vi "ReadConfig.vi"() -> ()   [LabVIEW 2021]
uses:
  <vilib>/Utility/file.llb/Read Delimited Spreadsheet (DBL).vi
panel:
  out "all rows":dbl[][](array[numeric])
  out "array":dbl[][](array[numeric])
  in  "text to write":string="test"
  out "error out":errorcluster
  out "text read":string
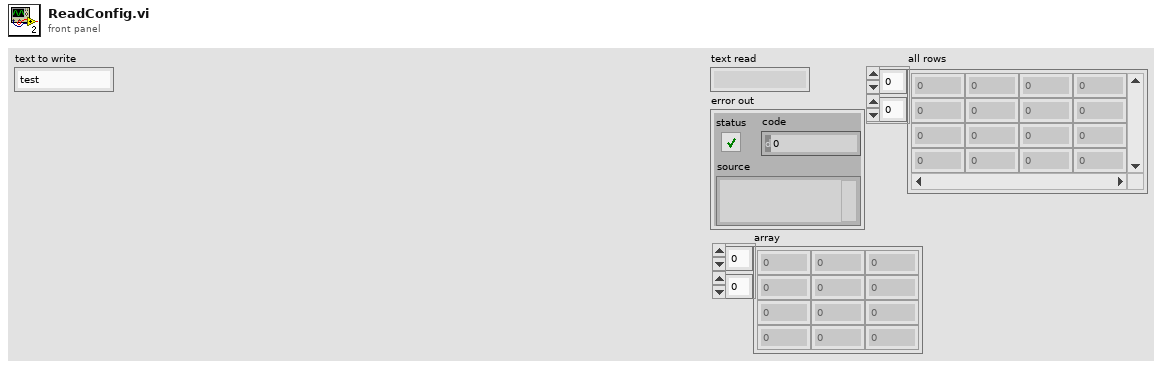
[diagram p1: front panel]
types:
  T1 = enum16{"open", "replace", "create", "open or create", "replace or create", "replace or create with confirmation"}
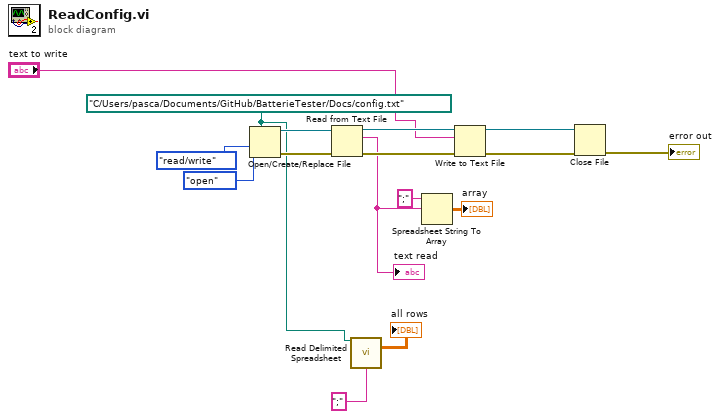
[diagram p0: block diagram]
diagram:
  w3 = path "C:/Users/pasca/Documents/GitHub/BatterieTester/Docs/config.txt"
  n1 = Open/Create/Replace File(file path (use dialog)=w3, operation (0:open)=T1."open", access (0:read/write)=enum16{"read/write", "read-only", "write-only"}."read/write") -> (refnum out=w14:refnum<file>, error out=w13:errorcluster)  [unwired: 3 in, 1 out]
  n2 = Read from Text File(file (use dialog)=w14, error in=w13) -> (refnum out=w9:refnum<file>, text=w6:string, error out=w12:errorcluster)  [unwired: 2 in, 1 out]
  "text read" <- w6
  n3 = call-poly <vilib>:"Read Delimited Spreadsheet.vi"("file path (dialog if empty)"=w3, "delimiter (\\t)"=";" ("delimiter (\\t)")) -> ("all rows"=→"all rows":dbl[][])  [unwired: 8 in, 5 out]
  n4 = Spreadsheet String To Array(format string=";", spreadsheet string=w6) -> (array=→"array":dbl[][])  [unwired: 2 in]
  n5 = Write to Text File(file (use dialog)=w9, text="text to write", error in=w12) -> (refnum out=w10:refnum<file>, error out=w11:errorcluster)  [unwired: 1 in, 1 out]
  n6 = Close File(refnum=w10, error in=w11) -> (error out=→"error out":errorcluster)  [unwired: 1 out]
